vi "(BASVR) Color Blank Channels White.vi"(10 "Channel # Column":i32[](array[numeric]), 11 "Channel Control & Legend":refnum<vi>) -> ()   [LabVIEW 2023]
uses:
  <vilib>/Utility/miscctls.llb/LVRowAndColumnTypeDef.ctl
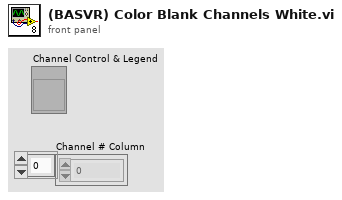
[diagram p1: front panel]
types:
  T1 = typedef "LVRowAndColumnTypeDef.ctl" = cluster{"Row":i32, "Column":i32}
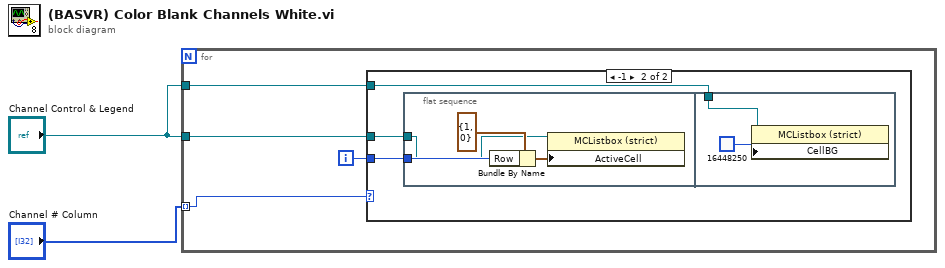
[diagram p0: block diagram]
diagram:
  n1 = for {
    tunnel: "Channel # Column" -> [w3] mode=indexing
    tunnel: "Channel Control & Legend" -> [w5]
    tunnel: "Channel Control & Legend" -> [w4]
    i -> [w6]
    n2 = case shown="-1" w3 {
      tunnel: w6 -> [_ w9]
      tunnel: w5 -> [_ w8]
      tunnel: w4 -> [_ w7]
      frame Default {
      }
      frame -1 {
        n3 = flat-sequence {
          tunnel: w9 -> [w12]
          tunnel: w8 -> [w10]
          tunnel: w7 -> [w14]
          frame #0 {
            n4 = Bundle By Name(cluster=T1 {"Row"=1, "Column"=0} ("Active Cell:Active Cell"), "Row"=w12) -> (w11:T1)
            n5 = property on="Property Node" class="MCListbox (strict)"(reference=w10, "ActiveCell"=w11) -> ()  [unwired: 1 in, 2 out]
          }
          frame #1 {
            n6 = property on="Property Node" class="MCListbox (strict)"(reference=w14, "CellBG"=u32 16448250) -> ()  [unwired: 1 in, 2 out]
          }
        }
      }
    }
  }
